vi "Initialize TCP Listen Resource.vi"(8 "error in (no error)":errorcluster, 11 "UR5 Robot in":refnum<class "UR5 Robot.lvclass">) -> (0 "error out":errorcluster, 3 "UR5 Robot out":refnum<class "UR5 Robot.lvclass">)   [LabVIEW 2018, in "UR5 Robot.lvlib" / "UR5 Robot.lvclass"]
uses:
  UR5 Robot.lvclass
  UR5 Robot.lvclass/UR5 Robot.ctl
  C:/AME Test Engineering/LabVIEW/PPLs/Robot/Parent/Robot.lvlibp/Robot.lvclass
  PPLs/Robot/Parent/Robot.lvlibp/Robot.lvclass
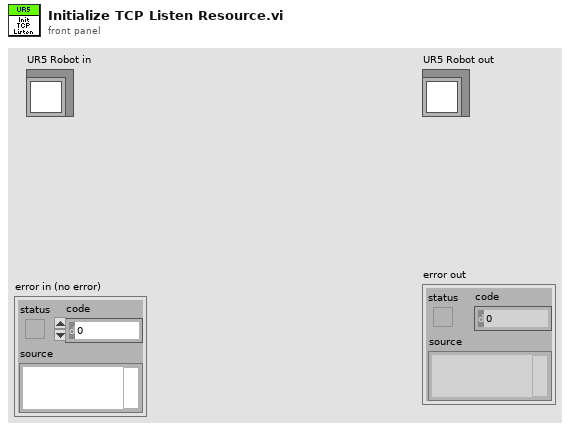
[diagram p1: front panel]
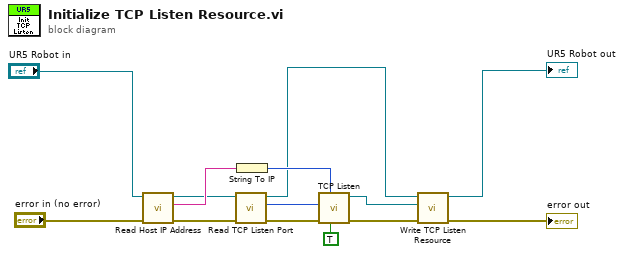
[diagram p0: block diagram]
diagram:
  n1 = call "Read Host IP Address.vi"("error in (no error)"="error in (no error)", "Robot in"="UR5 Robot in") -> ("error out"=w4:errorcluster, "Host IP Address"=w7:string, "Robot out"=w5:refnum<class "UR5 Robot.lvclass">)  [unwired: 7 in]
  n2 = call "Read TCP Listen Port.vi"("error in (no error)"=w4, "Robot in"=w5) -> ("error out"=w3:errorcluster, "TCP Listen Port"=w2:u16, "Robot out"=w1:refnum<class "UR5 Robot.lvclass">)  [unwired: 7 in]
  n3 = String To IP(1:w7) -> (0:w13:u32)
  n4 = call <vilib>:"TCP Listen.vi"("resolve remote address (T)"=TRUE, "net address"=w13, "error in (no error)"=w3, "port"=w2) -> ("error out"=w11:errorcluster, "connection ID"=w12:refnum<k5>)  [unwired: 3 in, 3 out]
  n5 = call "Write TCP Listen Resource.vi"("error in (no error)"=w11, "TCP Listen Resource"=w12, "UR5 Robot in"=w1) -> ("error out"=→"error out":errorcluster, "UR5 Robot out"=→"UR5 Robot out":refnum<class "UR5 Robot.lvclass">)  [unwired: 7 in]
